vi "logic-gates.vi"() -> ()   [LabVIEW 2025]
panel:
  out "Boolean 3":bool
  in  "Boolean 2":bool
  in  "Boolean":bool
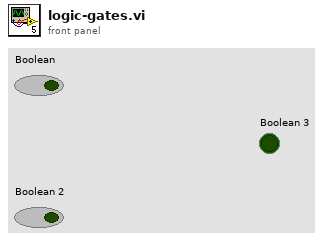
[diagram p1: front panel]
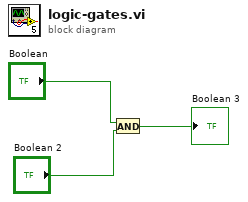
[diagram p0: block diagram]
diagram:
  n1 = And(x="Boolean", y="Boolean 2") -> (x .and. y?=→"Boolean 3":bool)
